vi "Run_Init Core.vi"(0 "Assignment Statement in":refnum<class "Assignment Statement.lvclass">, 11 "error in (no error)":errorcluster) -> (4 "Assignment Statement out":refnum<class "Assignment Statement.lvclass">, 15 "error out":errorcluster)   [LabVIEW 2016, in "Assignment Statement.lvclass"]
uses:
  Assignment Statement.lvclass
  E:/Repository/LabVIEW Script Language/source code/LSL components/functions/functionsbase/functionbase.lvclass
  functionsbase/functionbase.lvclass/functionbase.ctl
  functionsbase/functionbase.lvclass
  functionsbase/properties/Read RT Variables.vi
  variables/RT Variables/RT Variables.lvclass
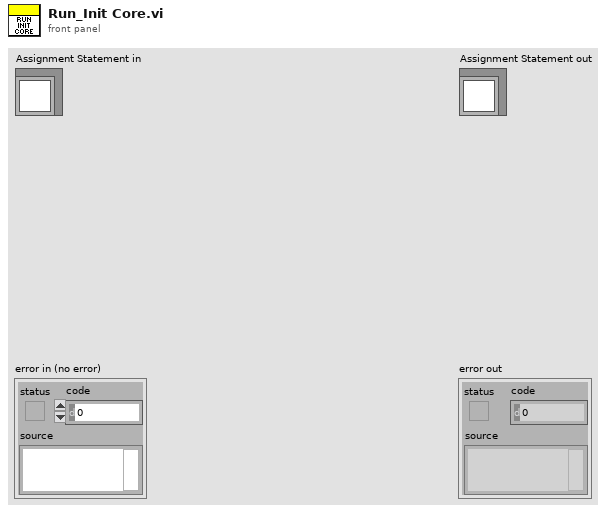
[diagram p1: front panel]
types:
  T1 = typedef "Datatype.ctl" = enum16{"Null", "Numeric", "String", "Bool", "Numeric 1D", "String 1D", "Bool 1D", "Numeric 2D", "String 2D", "Bool 2D", "Variant"}
  T2 = typedef "Valuetype.ctl" = enum16{"Value", "Variable", "Function"}
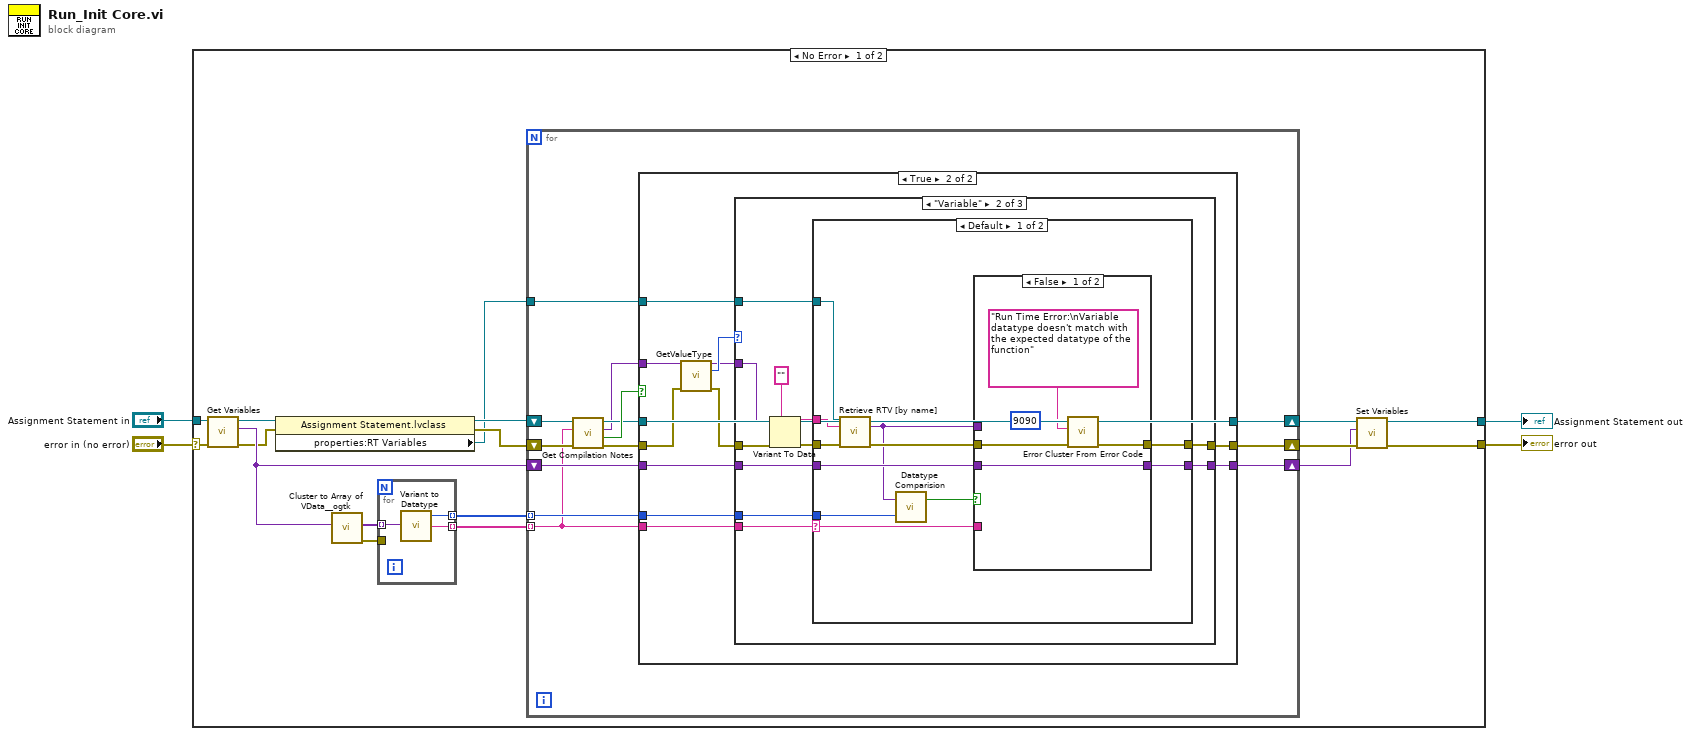
[diagram p0: block diagram]
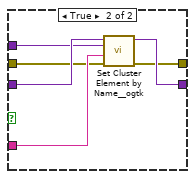
[diagram p4: hidden frame]
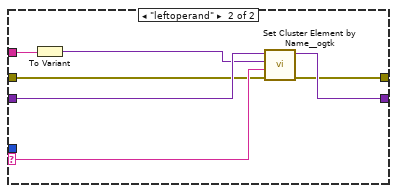
[diagram p5: hidden frame]
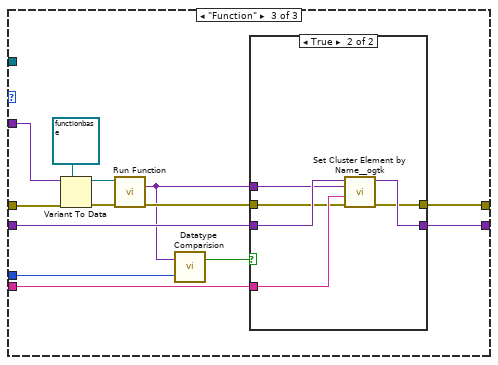
[diagram p6: hidden frame]
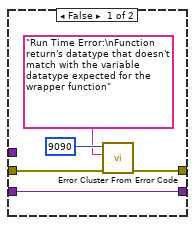
[diagram p7: hidden frame]
diagram:
  n1 = case shown="No Error" "error in (no error)" {
    selector: "error in (no error)" -> [w20 w120]
    tunnel: [w12 w120] -> w2
    tunnel: [w11 w119] -> w1
    tunnel: "Assignment Statement in" -> [w19 w119]
    frame No Error {
      n2 = call-dynamic "Get Variables.vi"("error in (no error)"=w20, "Message Popup in"=w19) -> ("error out"=w9:errorcluster, "Variables"=w16:variant, "Message Popup out"=w7:refnum<class "Assignment Statement.lvclass">)  [unwired: 7 in]
      n3 = property class="Assignment Statement.lvclass"(reference=w7, error in=w9) -> (reference out=w6:refnum<class "Assignment Statement.lvclass">, error out=w8:errorcluster, "properties:RT Variables"=w5:refnum<class "RT Variables.lvclass">)
      n4 = call <userlib>:"Cluster to Array of VData__ogtk.vi"("Cluster"=w16) -> ("error out"=w18:errorcluster, "Array of VData"=w21:variant[])  [unwired: 9 in]
      n5 = for {
        tunnel: w21 -> [w118] mode=indexing
        tunnel: [w117] -> w10 mode=indexing
        tunnel: [w116] -> w17 mode=indexing
        tunnel: w18 -> [_]
        n6 = call "Variant to Datatype.vi"("Variant"=w118) -> ("Name"=w116:string, "Datatype"=w117:T1)  [unwired: 2 in, 1 out]
      }
      n7 = for {
        shift-right: [w25] -> w15
        shift-left: w6 -> [w33]
        tunnel: w17 -> [w23] mode=indexing
        shift-right: [w31] -> w13
        shift-left: w16 -> [w32]
        shift-right: [w26] -> w14
        shift-left: w8 -> [w34]
        tunnel: w10 -> [w24] mode=indexing
        tunnel: w5 -> [w22]
        n8 = call "Get Compilation Notes.vi"("error in (no error)"=w34, "note key"=w23, "functionbase in"=w33) -> ("error out"=w28:errorcluster, "Found?"=w30:bool, "Notes"=w27:variant, "functionbase out"=w29:refnum<class "Assignment Statement.lvclass">)  [unwired: 5 in]
        n9 = case shown="True" w30 {
          tunnel: w32 -> [w35 w43]
          tunnel: [w35 w44] -> w31
          tunnel: w29 -> [w37 w49]
          tunnel: w28 -> [w36 w47]
          tunnel: w27 -> [_ w48]
          tunnel: [w36 w42] -> w26
          tunnel: [w37 w49] -> w25
          tunnel: w24 -> [_ w40]
          tunnel: w23 -> [_ w39]
          tunnel: w22 -> [_ w38]
          frame False {
          }
          frame True {
            n10 = call "GetValueType.vi"("variant"=w48, "error in"=w47) -> ("variant out"=w45:variant, "Value Type"=w46:T2, "error out"=w41:errorcluster)  [unwired: 11 in]
            n11 = case shown="\"Variable\"" w46 {
              tunnel: w45 -> [_ w61 w103]
              tunnel: [w51 w56 w99] -> w44
              tunnel: w43 -> [w51 w57 w100]
              tunnel: [w50 w55 w96] -> w42
              tunnel: w41 -> [w50 w62 w104]
              tunnel: w40 -> [_ w54 w94]
              tunnel: w39 -> [_ w53 w98]
              tunnel: w38 -> [_ w52 _]
              frame "Value", Default {
              }
              frame "Variable" {
                n12 = Variant To Data(error in=w62, type="", Variant=w61) -> (data=w58:string, error out=w59:errorcluster)
                n13 = case shown="Default" w53 {
                  selector: w53 -> [w68 w88]
                  tunnel: w59 -> [w73 w87]
                  tunnel: w58 -> [w65 w86]
                  tunnel: w57 -> [w72 w91]
                  tunnel: [w71 w90] -> w56
                  tunnel: [w70 w89] -> w55
                  tunnel: w54 -> [w67 _]
                  tunnel: w52 -> [w63 _]
                  frame Default {
                    n14 = call-dynamic "Retrieve RTV [by name].vi"("RT Variables in"=w63, "RTV name"=w65, "error in (no error)"=w73) -> ("Data"=w64:variant, "error out"=w69:errorcluster)  [unwired: 8 in, 3 out]
                    n15 = call "Datatype Comparision.vi"("Required Datatype"=w67, "Data"=w64) -> ("Equal?"=w66:bool)  [unwired: 1 in]
                    n16 = case shown="False" w66 {
                      tunnel: w72 -> [w78 w84]
                      tunnel: [w78 w83] -> w71
                      tunnel: w64 -> [_ w82]
                      tunnel: w68 -> [_ w81]
                      tunnel: w69 -> [w77 w80]
                      tunnel: [w76 w79] -> w70
                      frame False {
                        n17 = call <vilib>:"Error Cluster From Error Code.vi"("error in (no error)"=w77, "error message (\"\")"="Run Time Error:\nVariable datatype doesn't match with the expected datatype of the function" ("error message (\"\")"), "error code (0)"=9090) -> ("error out"=w76:errorcluster)  [unwired: 6 in]
                      }
                      frame True {
                        n18 = call <userlib>:"Set Cluster Element by Name__ogtk.vi"("error in (no error)"=w80, "Element Name (\"\": New Element Data Name)"=w81, "New Element Value"=w82, "Cluster"=w84) -> ("error out"=w79:errorcluster, "VCluster out"=w83:variant)  [unwired: 5 in, 1 out]
                      }
                    }
                  }
                  frame "leftoperand" {
                    n19 = To Variant(anything=w86) -> (Variant=w85:variant)
                    n20 = call <userlib>:"Set Cluster Element by Name__ogtk.vi"("error in (no error)"=w87, "Element Name (\"\": New Element Data Name)"=w88, "New Element Value"=w85, "Cluster"=w91) -> ("error out"=w89:errorcluster, "VCluster out"=w90:variant)  [unwired: 5 in, 1 out]
                  }
                }
              }
              frame "Function" {
                n21 = Variant To Data(error in=w104, type=refnum<class "functionbase.lvclass"> refnum ("functionbase.lvclass"), Variant=w103) -> (data=w92:refnum<class "functionbase.lvclass">, error out=w101:errorcluster)
                n22 = call-dynamic "Run Function.vi"("functionbase in"=w92, "error in (no error)"=w101) -> ("Return"=w95:variant, "error out"=w97:errorcluster)  [unwired: 11 in, 1 out]
                n23 = call "Datatype Comparision.vi"("Required Datatype"=w94, "Data"=w95) -> ("Equal?"=w93:bool)  [unwired: 1 in]
                n24 = case shown="True" w93 {
                  tunnel: w100 -> [w109 w115]
                  tunnel: [w109 w114] -> w99
                  tunnel: w95 -> [_ w113]
                  tunnel: w98 -> [_ w112]
                  tunnel: w97 -> [w108 w111]
                  tunnel: [w107 w110] -> w96
                  frame False {
                    n25 = call <vilib>:"Error Cluster From Error Code.vi"("error in (no error)"=w108, "error message (\"\")"="Run Time Error:\nFunction return's datatype that doesn't match with the variable datatype expected for the wrapper function" ("error message (\"\")"), "error code (0)"=9090) -> ("error out"=w107:errorcluster)  [unwired: 6 in]
                  }
                  frame True {
                    n26 = call <userlib>:"Set Cluster Element by Name__ogtk.vi"("error in (no error)"=w111, "Element Name (\"\": New Element Data Name)"=w112, "New Element Value"=w113, "Cluster"=w115) -> ("error out"=w110:errorcluster, "VCluster out"=w114:variant)  [unwired: 5 in, 1 out]
                  }
                }
              }
            }
          }
        }
      }
      n27 = call-dynamic "Set Variables.vi"("error in (no error)"=w14, "Variables"=w13, "Message Popup in"=w15) -> ("error out"=w12:errorcluster, "Message Popup out"=w11:refnum<class "Assignment Statement.lvclass">)  [unwired: 7 in]
    }
    frame Error {
    }
  }
  "error out" <- w2
  "Assignment Statement out" <- w1
